vi "Initialize Registers.vi"   [LabVIEW 2014]
uses:
  <vilib>/rvi/Emulation/niFpgaEmulationIsFPGAContextNoSignature.vi
  <vilib>/rvi/DataTransferAndStorage/Container/Common/niFpgaContainerGetUniqueNameForEmu.vi
  <vilib>/rvi/Memory/Memory_Emulation/niFpgaMemoryEmulationCacheClearOnFirstRun.vi
  <vilib>/rvi/Memory/Memory_Emulation/nirvimemoryEmulationManagerCache_MakeExclusive.vi
  <vilib>/rvi/Memory/Memory_Emulation/niFpgaMemoryEmulationValidateCache.vi
  <vilib>/rvi/Memory/Memory_Emulation/nirvimemoryEmulationManagerCache_InsertValue.vi
  <vilib>/Utility/error.llb/Clear Errors.vi
  <vilib>/rvi/Memory/Memory_Emulation/nirvimemoryEmulationManagerCache_ReleaseExclusive.vi
  <vilib>/rvi/Memory/Memory_Emulation/nirvimemoryEmulationManagerCache_GetValue.vi
  <vilib>/rvi/Memory/Memory_Emulation/nirvimemoryEmulationManagerCache_SetValue.vi
  <vilib>/rvi/Emulation/niFpgaProcessEmulError.vi
  <vilib>/rvi/Emulation/niFpgaSctlEmulationGetInTimedLoop.vi
  <vilib>/rvi/DataTransferAndStorage/Container/XNode/niFpgaContainer.xnode
  <vilib>/rvi/DataTransferAndStorage/Register/Emulation/niFpgaRegisterEmulation.vi
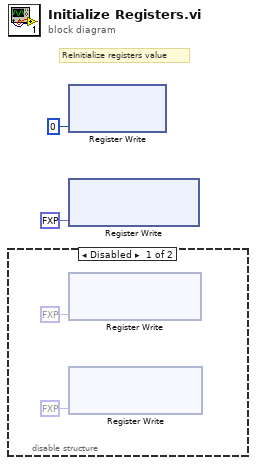
[diagram p0: block diagram]
diagram:
  # "ReInitialize registers value"
  n1 = disable-structure shown="Disabled" {
    frame Disabled {
      n2 = xnode ("Register Write")("Data"=fxp<+,44,44> 0.0) -> ()  [unwired: 1 in, 1 out]
      n3 = xnode ("Register Write")("Data"=fxp<+,44,44> 0.0) -> ()  [unwired: 1 in, 1 out]
    }
    frame Enabled {
    }
  }
  n4 = xnode ("Register Write")("Data"=0) -> ()  [unwired: 1 in, 1 out]
  n5 = xnode ("Register Write")("Data"=fxp<+,44,44> 0.0) -> ()  [unwired: 1 in, 1 out]
